vi "Ke2000 Configure DC Current.vi"(4 "Digital Filter Readings (10)":i32=10, 5 "Resolution (7: 6.5 digits)":u16(ring)=7 items=["3.5 Digits"=4, "4.5 Digits"=5, "5.5 Digits"=6, "6.5 Digits"=7], 6 "Digital Filter (0: Off)":u16(ring) items=["Off", "Moving Filter", "Repeating Filter"], 7 "Auto Range? (T: Auto)":bool=TRUE, 8 "error in":errorcluster, 10 "Custom Range (0 A)":dbl format="%#_6p", 11 "VISA resource name":refnum<visa-resource-name>) -> (0 "error out":errorcluster, 3 "VISA resource name out":refnum<visa-resource-name>)   [LabVIEW 2017]
panel:
  out "Error Messages":string
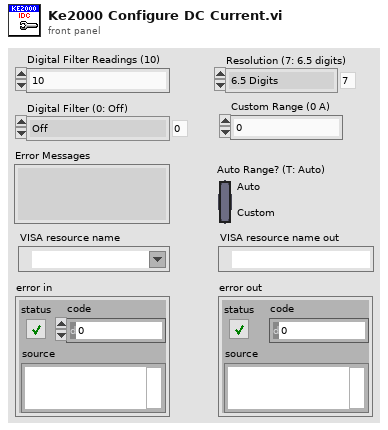
[diagram p1: front panel]
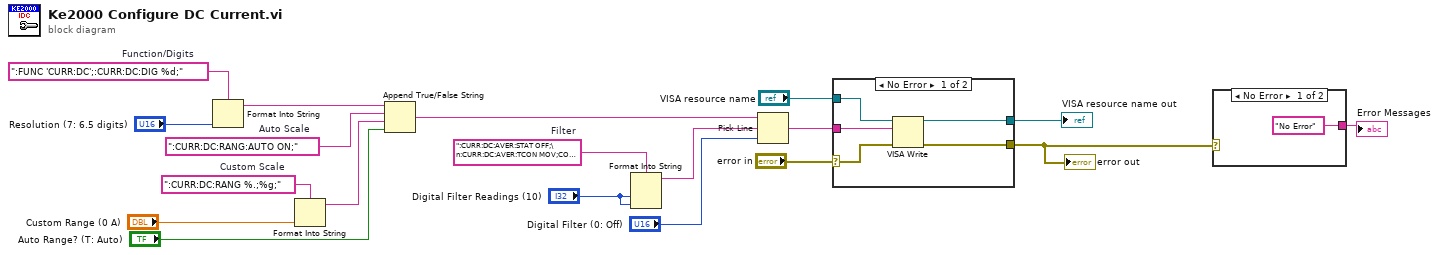
[diagram p0: block diagram]
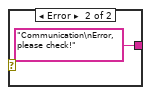
[diagram p2: hidden frame]
diagram:
  w11 = ":CURR:DC:AVER:STAT OFF;\n:CURR:DC:AVER:TCON MOV;COUN %d;STAT ON;\n:CURR:DC:AVER:TCON REP;COUN %d;STAT ON;"  # Filter
  w17 = ":CURR:DC:RANG %.;%g;"  # Custom Scale
  w14 = ":CURR:DC:RANG:AUTO ON;"  # Auto Scale
  w19 = ":FUNC 'CURR:DC';:CURR:DC:DIG %d;"  # Function/Digits
  n1 = Format Into String(format string=w19, "Resolution (7: 6.5 digits)") -> (resulting string=w13:string)  [unwired: 2 in, 1 out]
  n2 = Format Into String(format string=w17, "Custom Range (0 A)") -> (resulting string=w15:string)  [unwired: 2 in, 1 out]
  n3 = Append True/False String(1:"Auto Range? (T: Auto)", 2:w15, 3:w14, 4:w13) -> (0:w9:string)
  n4 = Format Into String(format string=w11, "Digital Filter Readings (10)", "Digital Filter Readings (10)") -> (resulting string=w8:string)  [unwired: 2 in, 1 out]
  n5 = Pick Line(string ("")=w9, multi-line string=w8, line index="Digital Filter (0: Off)") -> (output string=w6:string)
  n6 = case shown="No Error" "error in" {
    selector: "error in" -> [w22 w26]
    tunnel: w6 -> [w24 _]
    tunnel: "VISA resource name" -> [w23 w25]
    tunnel: [w21 w26] -> w2
    tunnel: [w20 w25] -> w3
    frame No Error {
      n7 = VISA Write(VISA resource name=w23, write buffer=w24, error in (no error)=w22) -> (VISA resource name out=w20:refnum<visa-resource-name>, error out=w21:errorcluster)  [unwired: 1 out]
    }
    frame Error {
    }
  }
  "error out" <- w2
  "VISA resource name out" <- w3
  n8 = case shown="No Error" w2 {
    tunnel: ["No Error" "Communication\nError, please check!"] -> w1
    frame No Error {
    }
    frame Error {
    }
  }
  "Error Messages" <- w1
